vi "SystemsCheckPressureLimitGLOBAL.vi"() -> ()   [LabVIEW 2017]
panel:
  in  "Magnetic Pressure Limit (PSI)":dbl=70.0
  in  "Suspension Pressure Limit (PSI)":dbl=70.0
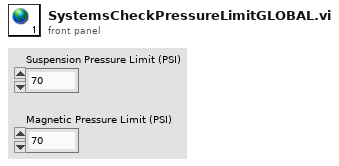
[diagram p1: front panel]
diagram:
